vi "BMP180 Read.vi"(8 "error in (no error)":errorcluster, 9 "BMP180 Config":T1={"I2C"={"Slave Address"=64, "Channel"=0}, "Mode"=enum."Ultra Low Power", "Cal Coefs"={"AC1"={"Addr:"=170, "Val:"=0}, "AC2"={"Addr:"=172, "Val:"=0}, "AC3"={"Addr:"=174, "Val:"=0}, "AC4"={"Addr:"=176, "Val:"=0}, "AC5"={"Addr:"=178, "Val:"=0}, "AC6"={"Addr:"=180, "Val:"=0}, "B1"={"Addr:"=182, "Val:"=0}, "B2"={"Addr:"=184, "Val:"=0}, "MB"={"Addr:"=186, "Val:"=0}, "MC"={"Addr:"=188, "Val:"=0}, "MD"={"Addr:"=190, "Val:"=0}}} {"I2C"."Slave Address" format="%.0x"; "Cal Coefs"."MD"."Val:" format="%04x"; "Cal Coefs"."MD"."Addr:" format="%02x"; "Cal Coefs"."MC"."Val:" format="%04x"; "Cal Coefs"."MC"."Addr:" format="%02x"; "Cal Coefs"."MB"."Val:" format="%04x"; "Cal Coefs"."MB"."Addr:" format="%02x"; "Cal Coefs"."B2"."Val:" format="%04x"; "Cal Coefs"."B2"."Addr:" format="%02x"; "Cal Coefs"."B1"."Val:" format="%04x"; "Cal Coefs"."B1"."Addr:" format="%02x"; "Cal Coefs"."AC6"."Val:" format="%04x"; "Cal Coefs"."AC6"."Addr:" format="%02x"; "Cal Coefs"."AC5"."Val:" format="%04x"; "Cal Coefs"."AC5"."Addr:" format="%02x"; "Cal Coefs"."AC4"."Val:" format="%04x"; "Cal Coefs"."AC4"."Addr:" format="%02x"; "Cal Coefs"."AC3"."Val:" format="%04x"; "Cal Coefs"."AC3"."Addr:" format="%02x"; "Cal Coefs"."AC2"."Val:" format="%04x"; "Cal Coefs"."AC2"."Addr:" format="%02x"; "Cal Coefs"."AC1"."Val:" format="%04x"; "Cal Coefs"."AC1"."Addr:" format="%02x"}, 11 "LINX Resource in":T2) -> (0 "error out":errorcluster, 1 "Temperature (F)":dbl, 2 "Temperature (C)":dbl, 3 "LINX Resource":T2, 5 "Pressure":i32 format="%.0f Pa")   [LabVIEW 2014]
uses:
  <vilib>/MakerHub/LINX/Private/Type Defs/LINX Ref.ctl
  <vilib>/MakerHub/LINX/Private/Type Defs/Platform.ctl
  <vilib>/MakerHub/LINX/Private/Type Defs/Interface.ctl
  <vilib>/MakerHub/LINX/Private/Device/Type Defs/LINX Device Config.ctl
  <vilib>/MakerHub/LINX/Private/Device/Type Defs/TCP Config.ctl
  <vilib>/MakerHub/LINX/Private/Device/Type Defs/Channels.ctl
  BMP180 Config Options.ctl
  <vilib>/MakerHub/LINX/LMH-LINX.lvlib
  <vilib>/MakerHub/LINX/Private/Device/Device.lvlib
panel:
  out "Raw Pres":i32
  out "Raw Temp":i32
  out "B6":i32
  out "B7":u32
  out "B4":u32
  out "B3":i32
  out "B5":i32
  out "X3":i32
  out "X2":i32
  out "X1":i32
  # "These values are solely for checking work"
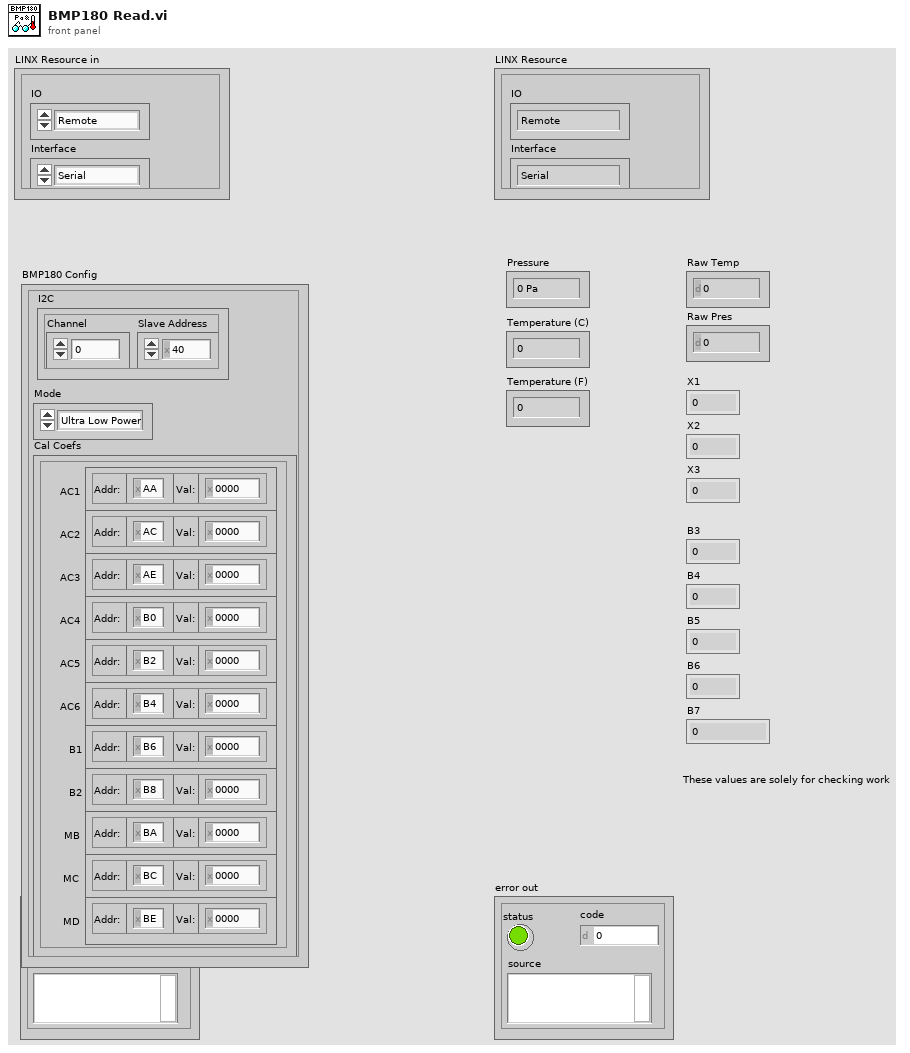
[diagram p1: front panel]
types:
  T1 = typedef "BMP180 Config Options.ctl" = cluster{"I2C":cluster{"Slave Address":u8, "Channel":u8}, "Mode":enum8{"Ultra Low Power", "Standard", "High Resolution", "Ultra High Resolution"}, "Cal Coefs":cluster{"AC1":cluster{"Addr:":u8, "Val:":u16}, "AC2":cluster{"Addr:":u8, "Val:":u16}, "AC3":cluster{"Addr:":u8, "Val:":u16}, "AC4":cluster{"Addr:":u8, "Val:":u16}, "AC5":cluster{"Addr:":u8, "Val:":u16}, "AC6":cluster{"Addr:":u8, "Val:":u16}, "B1":cluster{"Addr:":u8, "Val:":u16}, "B2":cluster{"Addr:":u8, "Val:":u16}, "MB":cluster{"Addr:":u8, "Val:":u16}, "MC":cluster{"Addr:":u8, "Val:":u16}, "MD":cluster{"Addr:":u8, "Val:":u16}}}
  T2 = typedef "LMH-LINX.lvlib/LINX Ref.ctl" = cluster{"IO":T3, "Interface":T4, "LINX Device Config":T5}
  T3 = typedef "LMH-LINX.lvlib/Platform.ctl" = enum16{"Remote", "Local"}
  T4 = typedef "LMH-LINX.lvlib/Interface.ctl" = enum16{"Serial", "TCP"}
  T5 = typedef "LMH-LINX.lvlib/Device.lvlib/LINX Device Config.ctl" = cluster{"Interface":T4, "COM Port":refnum<visa-resource-name>, "TCP Configuration":T6, "Device Family":u8, "Device ID":u8, "Device Name":string, "TCP Ref":refnum<k5>, "Channels":T7}
  T6 = typedef "LMH-LINX.lvlib/Device.lvlib/TCP Config.ctl" = cluster{"IP Address":string, "Port":u16}
  T7 = typedef "LMH-LINX.lvlib/Channels.ctl" = cluster{"DI":u8[], "DO":u8[], "AI":u8[], "AO":u8[], "PWM":u8[], "QE":u8[], "UART":u8[], "I2C 2":u8[], "SPI":u8[], "CAN":u8[], "Servo":u8[], "AI Ref (V)":dbl, "AI Resolution (Bits)":u8, "AO Ref (V)":dbl, "AO Resolution (Bits)":u8}
  T8 = enum8{"Ultra Low Power", "Standard", "High Resolution", "Ultra High Resolution"}
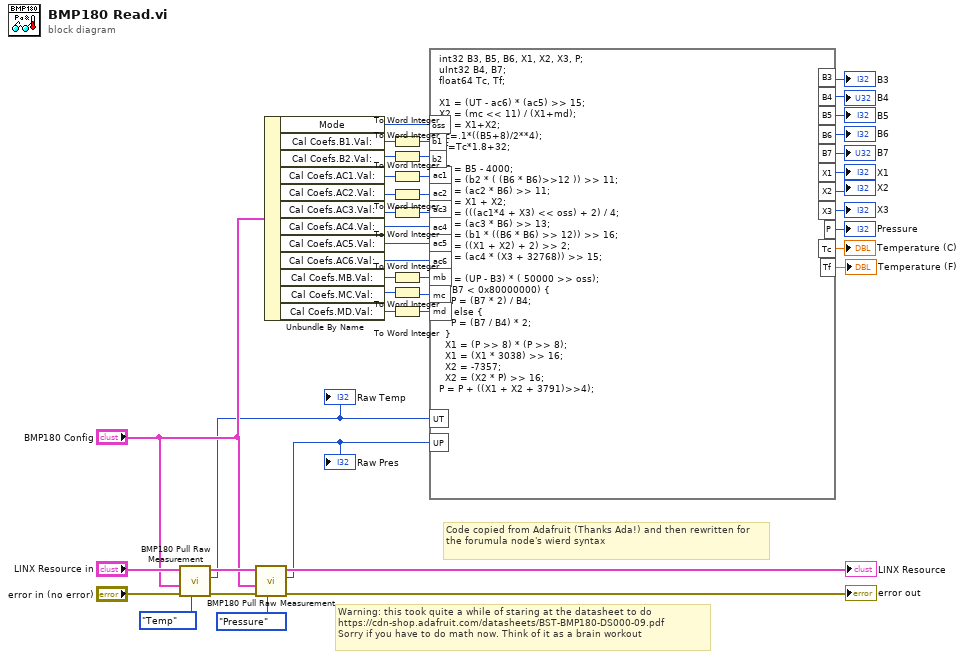
[diagram p0: block diagram]
diagram:
  # "Code copied from Adafruit (Thanks Ada!) and then rewritten for the forumula node's wierd syntax"
  # "Warning: this took quite a while of staring at the datasheet to do\nhttps://cdn-shop.adafruit.com/datasheets/BST-BMP180-DS000-09.pdf\nSorry if you have to do math now. Think of it as a brain workout"
  n1 = call "BMP180 Pull Raw Measurement.vi"("Sensor Type"=enum16{"Temp", "Pressure"}."Temp", "error in (no error)"="error in (no error)", "BMP180 Config"="BMP180 Config", "LINX Resource in"="LINX Resource in") -> ("error out"=w38:errorcluster, "Raw Reading"=w2:i32, "LINX Resource"=w39:T2)  [unwired: 5 in]
  "Raw Temp" <- w2
  n2 = call "BMP180 Pull Raw Measurement.vi"("Sensor Type"=enum16{"Temp", "Pressure"}."Pressure", "error in (no error)"=w38, "BMP180 Config"="BMP180 Config", "LINX Resource in"=w39) -> ("error out"=→"error out":errorcluster, "Raw Reading"=w1:i32, "LINX Resource"=→"LINX Resource":T2)  [unwired: 5 in]
  "Raw Pres" <- w1
  n3 = Unbundle By Name("BMP180 Config") -> ("Mode"=w21:T8, "Cal Coefs.B1.Val:"=w22:u16, "Cal Coefs.B2.Val:"=w19:u16, "Cal Coefs.AC1.Val:"=w18:u16, "Cal Coefs.AC2.Val:"=w17:u16, "Cal Coefs.AC3.Val:"=w16:u16, "Cal Coefs.AC4.Val:"=w15:u16, "Cal Coefs.AC5.Val:"=w14:u16, "Cal Coefs.AC6.Val:"=w13:u16, "Cal Coefs.MB.Val:"=w24:u16, "Cal Coefs.MC.Val:"=w10:u16, "Cal Coefs.MD.Val:"=w23:u16)
  n4 = To Word Integer(number=w22) -> (16bit integer=w20:i16)
  n5 = To Word Integer(number=w19) -> (16bit integer=w28:i16)
  n6 = To Word Integer(number=w18) -> (16bit integer=w27:i16)
  n7 = To Word Integer(number=w17) -> (16bit integer=w26:i16)
  n8 = To Word Integer(number=w16) -> (16bit integer=w25:i16)
  n9 = To Word Integer(number=w24) -> (16bit integer=w12:i16)
  n10 = To Word Integer(number=w10) -> (16bit integer=w11:i16)
  n11 = To Word Integer(number=w23) -> (16bit integer=w9:i16)
  n12 = formula code="int32 B3, B5, B6, X1, X2, X3, P;\nuInt32 B4, B7;\nfloat64 Tc, Tf;\n\nX1 = (UT - ac6) * (ac5) >> 15;\nX2 = (mc << 11) / (X1+md);\nB5 = X1+X2;\nTc=.1*((B5+8)/2**4);\nTf=Tc*1.8+32;\n\nB6 = B5 - 4000;\nX1 = (b2 * ( (B6 * B6)>>12 )) >> 11;\nX2 = (ac2 * B6) >> 11;\nX3 = X1 + X2;\nB3 = (((ac1*4 + X3) << oss) + 2) / 4;\nX1 = (ac3 * B6) >> 13;\nX2 = (b1 * ((B6 * B6) >> 12)) >> 16;\nX3 = ((X1 + X2) + 2) >> 2;\nB4 = (ac4 * (X3 + 32768)) >> 15;\n  \nB7 = (UP - B3) * ( 50000 >> oss);\nif (B7 < 0x80000000) {\n    P = (B7 * 2) / B4;\n  } else {\n    P = (B7 / B4) * 2;\n  }\n  X1 = (P >> 8) * (P >> 8);\n  X1 = (X1 * 3038) >> 16;\n  X2 = -7357; \n  X2 = (X2 * P) >> 16;\nP = P + ((X1 + X2 + 3791)>>4);"("UT"=w2, "ac1"=w27, "ac2"=w26, "ac3"=w25, "ac4"=w15, "b2"=w28, "b1"=w20, "oss"=w21, "UP"=w1, "ac5"=w14, "ac6"=w13, "mb"=w12, "mc"=w11, "md"=w9) -> ("P"=→"Pressure":i32, "X1"=→"X1":i32, "X2"=→"X2":i32, "B5"=→"B5":i32, "B3"=→"B3":i32, "B4"=→"B4":u32, "B6"=→"B6":i32, "X3"=→"X3":i32, "Tc"=→"Temperature (C)":dbl, "B7"=→"B7":u32, "Tf"=→"Temperature (F)":dbl)
